vi "检索模块.vi"(3 "错误输入":errorcluster caption="错误输入（无错误）", 4 "检索参数配置输入":T2={"发送指令"="+TXYBJT TECH", "等待时间（毫秒）"=500, "响应数据"="DTU Software,VER", "波特率"=[1200, 2400, 4800, 9600, 19200]}, 5 "COM号":refnum<visa-resource-name>) -> (0 "错误输出":errorcluster, 1 "串口参数输出":T1={"COM号"="", "波特率"=9600, "数据比特"=8, "奇偶"=enum."None", "停止位"=10, "流控制"=0} {"流控制" items=["无"=0, "XON/XOFF"=1, "RTS/CTS"=2, "DTR/DSR"=4]; "停止位" items=["1.0"=10, "1.5"=15, "2.0"=20]; "波特率" items=["75"=75, "110"=110, "134"=134, "150"=150, "300"=300, "600"=600, "1200"=1200, "1800"=1800, "2400"=2400, "4800"=4800, "7200"=7200, "9600"=9600, "14400"=14400, "19200"=19200, "28800"=28800, "38400"=38400, "56000"=56000, "57600"=57600, "115200"=115200, "128000"=128000, "230400"=230400]}, 2 "isfind？":bool)   [LabVIEW 2015]
uses:
  Serial - Settings.ctl
  <vilib>/Instr/_visa.llb/VISA Flush IO Buffer Mask.ctl
  <vilib>/Instr/_visa.llb/VISA Configure Serial Port (Instr).vi
panel:
  out "当前波特率":u32
  out "延时时间":u32
  out "波特率":T3=[1200, 4800, 9600, 19200]
  out "响应数据":string
  out "发送指令":string
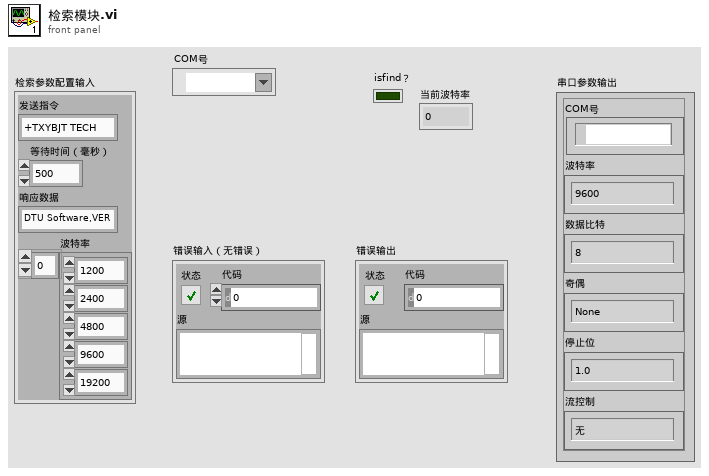
[diagram p1: front panel]
types:
  T1 = typedef "Serial - Settings.ctl" = cluster{"COM号":refnum<visa-resource-name>, "波特率":u32, "数据比特":u16, "奇偶":enum16{"None", "Odd", "Even", "Mark", "Space"}, "停止位":u16, "流控制":u16}
  T2 = typedef "检索模块.ctl" = cluster{"发送指令":string, "等待时间（毫秒）":u32, "响应数据":string, "波特率":T3}
  T3 = typedef "波特率.ctl" = u32[]
  T4 = typedef "VISA Flush IO Buffer Mask.ctl" = u16
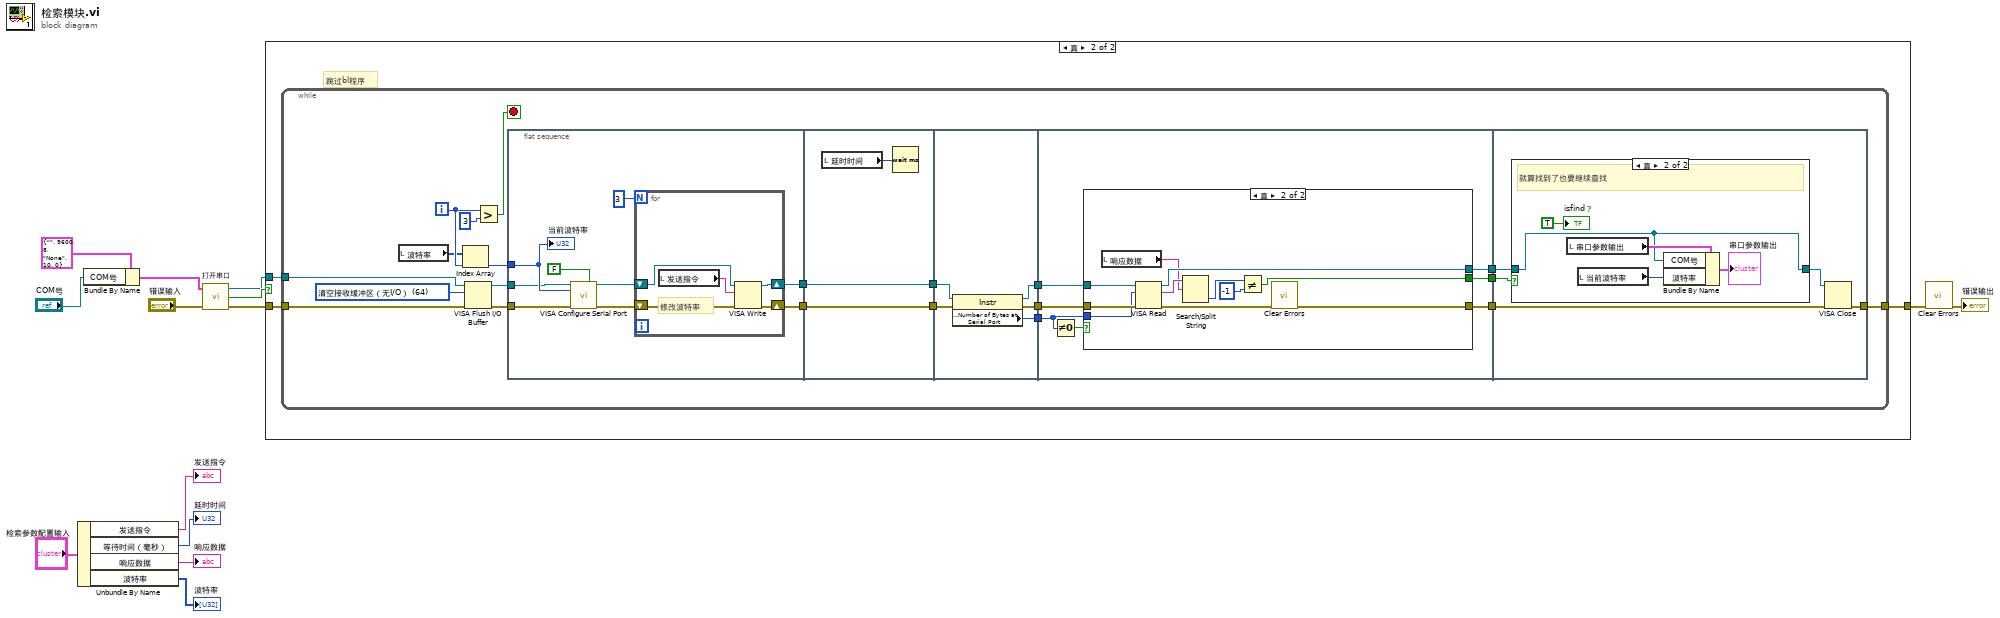
[diagram p0: block diagram]
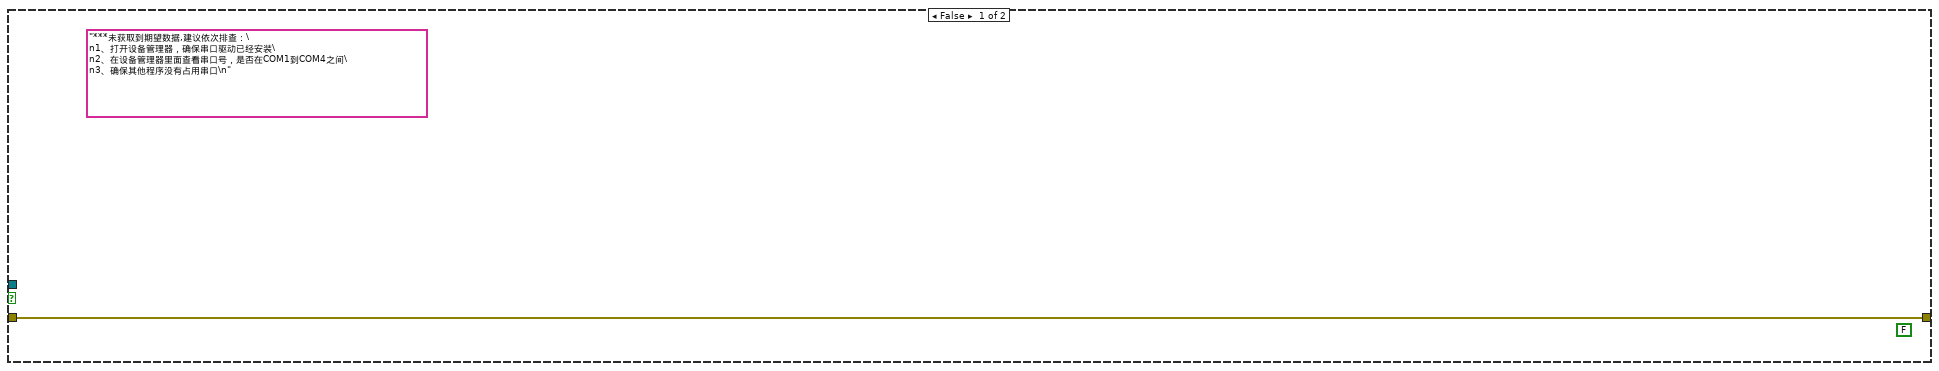
[diagram p2: hidden frame]
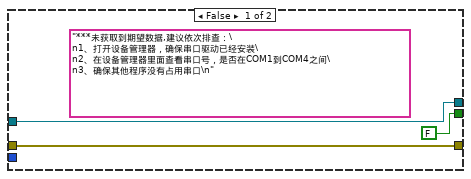
[diagram p3: hidden frame]
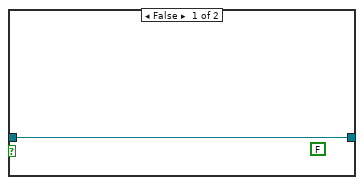
[diagram p4: hidden frame]
diagram:
  n1 = Unbundle By Name("检索参数配置输入") -> ("发送指令"=→"发送指令":string, "等待时间（毫秒）"=→"延时时间":u32, "响应数据"=→"响应数据":string, "波特率"=→"波特率":T3)
  n2 = Bundle By Name(cluster=T1 {"COM号"="", "波特率"=9600, "数据比特"=8, "奇偶"=enum."None", "停止位"=10, "流控制"=0} ("串口设置"), "COM号"="COM号") -> (w8:T1)
  n3 = call "打开串口.vi"("错误输入（无错误）"="错误输入", "串口设置"=w8) -> ("错误输出"=w10:errorcluster, "OpenOK?"=w13:bool, "VISA引用句柄输出"=w12:refnum<visa-resource-name>)  [unwired: 1 in]
  n4 = case shown="真" w13 {
    tunnel: w12 -> [_ w16]
    tunnel: w10 -> [w15 w17]
    tunnel: [w15 w18] -> w1
    frame False {
      (unwired) "***未获取到期望数据,建议依次排查：\n1、打开设备管理器，确保串口驱动已经安装\n2、在设备管理器里面查看串口号，是否在COM1到COM4之间\n3、确保其他程序没有占用串口\n" ("字符串 2")
      (unwired) FALSE
    }
    frame True {
      # "跳过bl程序"
      n5 = while {
        tunnel: w17 -> [w27]
        tunnel: [w34] -> w18
        tunnel: w16 -> [w20]
        i -> [w31]
        stop <- w19 stop-if-true
        w25 = T4 64 items=["清空接收缓冲区"=16, "向设备写入传输缓冲区"=32, "清空接收缓冲区（无I/O）"=64, "清空传输缓冲区"=128] ("Mask")
        n6 = local read "波特率"() -> (w24:T3)
        n7 = Index Array(array=w24, index=w31) -> (element=w39:u32)
        n8 = VISA Flush I/O Buffer(VISA resource name=w20, mask (16)=w25, error in (no error)=w27) -> (VISA resource name out=w28:refnum<visa-resource-name>, error out=w26:errorcluster)
        n9 = Greater?(x=w31, y=3) -> (0:w19:bool)
        n10 = flat-sequence {
          tunnel: w28 -> [w44]
          tunnel: w26 -> [w43]
          tunnel: w39 -> [w48]
          tunnel: [w46] -> w33
          tunnel: [w45] -> w32
          tunnel: w33 -> [w56]
          tunnel: w32 -> [w55]
          tunnel: [w55] -> w30
          tunnel: [w56] -> w29
          tunnel: [w59] -> w37
          tunnel: [w58] -> w36
          tunnel: [w57] -> w35
          tunnel: w30 -> [w61]
          tunnel: w29 -> [w60]
          tunnel: w37 -> [w66]
          tunnel: w36 -> [w65]
          tunnel: w35 -> [w67]
          tunnel: [w64] -> w23
          tunnel: [w63] -> w22
          tunnel: [w62] -> w21
          tunnel: [w83] -> w34
          tunnel: w23 -> [w87]
          tunnel: w22 -> [w84]
          tunnel: w21 -> [w86]
          frame #0 {
            n11 = call-poly "VISA Configure Serial Port"("VISA resource name"=w44, "Enable Termination\nChar (T)"=FALSE ("Enable Termination\nChar (T)"), "baud rate (9600)"=w48, "error in (no error)"=w43) -> ("VISA resource name out"=w42:refnum<visa-resource-name>, "error out"=w41:errorcluster)  [unwired: 10 in]
            n12 = for {
              N: 3 -> [_]
              shift-right: [w53] -> w46
              shift-left: w42 -> [w51]
              shift-right: [w52] -> w45
              shift-left: w41 -> [w50]
              # "修改波特率"
              n13 = local read "发送指令"() -> (w49:string)
              n14 = VISA Write(VISA resource name=w51, write buffer=w49, error in (no error)=w50) -> (VISA resource name out=w53:refnum<visa-resource-name>, error out=w52:errorcluster)  [unwired: 1 out]
            }
            "当前波特率" <- w48
          }
          frame #1 {
            n15 = local read "延时时间"() -> (w54:u32)
            n16 = Wait (ms)(milliseconds to wait=w54) -> ()  [unwired: 1 out]
          }
          frame #2 {
            n17 = property class="Instr"(reference=w60, error in=w61) -> (reference out=w59:refnum<visa-resource-name>, error out=w58:errorcluster, "Serial Settings:Number of Bytes at Serial Port"=w57:u32)
          }
          frame #3 {
            n18 = Not Equal To 0?(x=w67) -> (x != 0?=w68:bool)
            n19 = case shown="真" w68 {
              tunnel: [w70 w82] -> w63
              tunnel: w66 -> [w71 w74]
              tunnel: w65 -> [w70 w79]
              tunnel: [w71 w77] -> w64
              tunnel: w67 -> [_ w76]
              tunnel: [FALSE w75] -> w62
              frame False {
                (unwired) "***未获取到期望数据,建议依次排查：\n1、打开设备管理器，确保串口驱动已经安装\n2、在设备管理器里面查看串口号，是否在COM1到COM4之间\n3、确保其他程序没有占用串口\n" ("字符串 2")
              }
              frame True {
                n20 = local read "响应数据"() -> (w72:string)
                n21 = VISA Read(VISA resource name=w74, byte count=w76, error in (no error)=w79) -> (VISA resource name out=w77:refnum<visa-resource-name>, read buffer=w73:string, error out=w78:errorcluster)  [unwired: 1 out]
                n22 = Search/Split String(string=w73, search string/char (-)=w72) -> (offset of match=w81:i32)  [unwired: 1 in, 2 out]
                n23 = Not Equal?(x=w81, y=-1) -> (x != y?=w75:bool)
                n24 = call <vilib>:"Clear Errors.vi"("error in (no error)"=w78) -> ("error out"=w82:errorcluster)  [unwired: 5 in, 1 out]
              }
            }
          }
          frame #4 {
            n25 = case shown="真" w86 {
              tunnel: w87 -> [w88 w91]
              tunnel: [w88 w91] -> w85
              frame False {
                (unwired) FALSE ("T button?")
              }
              frame True {
                # "就算找到了也要继续查找"
                n26 = local read "串口参数输出"() -> (w93:T1)
                n27 = local read "当前波特率"() -> (w92:u32)
                n28 = Bundle By Name(cluster=w93, "COM号"=w91, "波特率"=w92) -> (→"串口参数输出":T1)
                "isfind？" <- TRUE ("T button?")
              }
            }
            n29 = VISA Close(VISA resource name=w85, error in (no error)=w84) -> (error out=w83:errorcluster)
          }
        }
      }
    }
  }
  n30 = call <vilib>:"Clear Errors.vi"("error in (no error)"=w1) -> ("error out"=→"错误输出":errorcluster)  [unwired: 5 in, 1 out]
